vi "daq+.vi"() -> ()   [LabVIEW 2020]
uses:
  <vilib>/Instr/_visa.llb/VISA Configure Serial Port (Instr).vi
panel:
  in  "Tab Control":enum32{"CONFIG", "DASHBOARD"}(tab)
  in  "stop":bool
  in  "Baudios":u32=9600
  in  "Paridad":enum16{"None", "Odd", "Even", "Mark", "Space"}(ring)
  in  "Puerto COM":refnum<visa-resource-name>
  out "ADC-dsPIC33FJ32MC202":dbl[](array[slide]) scale=0.0..4095.0
  in  "LED1":bool
  in  "LED2":bool
  in  "LED3":bool
  in  "LED4":bool
  out "error out":errorcluster
  out "VISA resource name out":refnum<visa-resource-name>
  out "read buffer":string
  # "CURSO DSPIC Y SUS APLICACIONES\nCLASE 5"
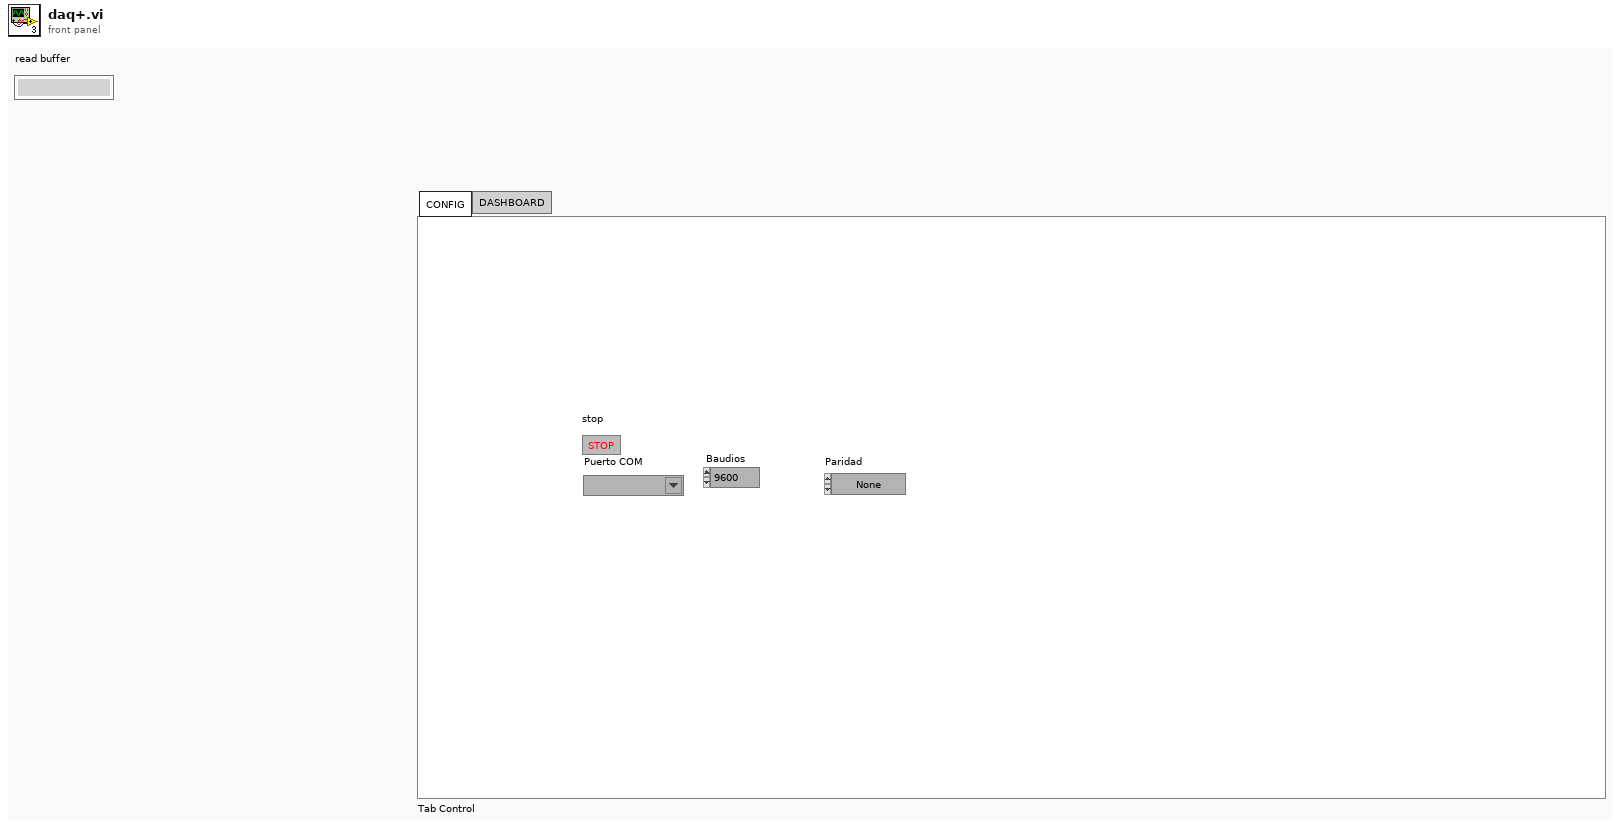
[diagram p1: front panel]
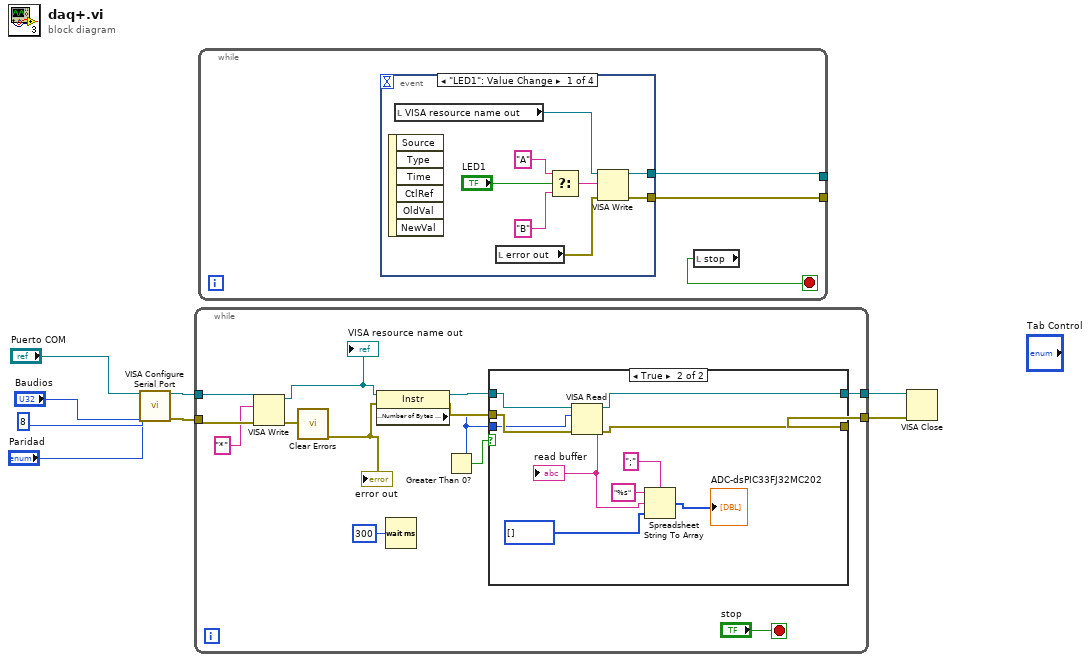
[diagram p0: block diagram]
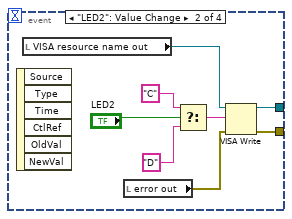
[diagram p2: hidden frame]
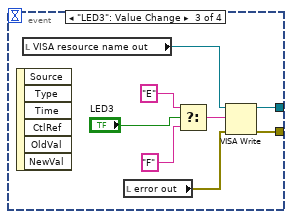
[diagram p3: hidden frame]
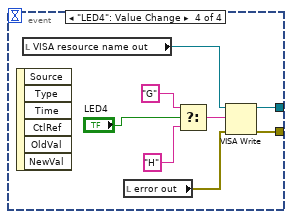
[diagram p4: hidden frame]
diagram:
  n1 = call-poly "VISA Configure Serial Port"("VISA resource name"="Puerto COM", "baud rate (9600)"="Baudios", "data bits (8)"=u16 8, "parity (0:none)"="Paridad") -> ("VISA resource name out"=w4:refnum<visa-resource-name>, "error out"=w3:errorcluster)  [unwired: 10 in]
  n2 = while {
    tunnel: w4 -> [w21]
    tunnel: w3 -> [w20]
    tunnel: [w14] -> w2
    tunnel: [w12] -> w1
    stop <- "stop" stop-if-true
    n3 = VISA Write(VISA resource name=w21, write buffer="*", error in (no error)=w20) -> (VISA resource name out=w9:refnum<visa-resource-name>, error out=w10:errorcluster)  [unwired: 1 out]
    "VISA resource name out" <- w9
    n4 = call <vilib>:"Clear Errors.vi"("error in (no error)"=w10) -> ("error out"=w11:errorcluster)  [unwired: 5 in, 1 out]
    "error out" <- w11
    n5 = property class="Instr"(reference=w9, error in=w11) -> (reference out=w17:refnum<visa-resource-name>, error out=w16:errorcluster, "Serial Settings:Number of Bytes at Serial Port"=w15:u32)
    n6 = Wait (ms)(milliseconds to wait=u32 300) -> ()  [unwired: 1 out]
    n7 = Greater Than 0?(x=w15) -> (x > 0?=w18:bool)
    n8 = case shown="True" w18 {
      tunnel: w17 -> [w24 w34]
      tunnel: w16 -> [w23 w33]
      tunnel: w15 -> [_ w32]
      tunnel: [w24 w26] -> w14
      tunnel: [w23 w25] -> w12
      frame False {
      }
      frame True {
        n9 = VISA Read(VISA resource name=w34, byte count=w32, error in (no error)=w33) -> (VISA resource name out=w26:refnum<visa-resource-name>, read buffer=w29:string, error out=w25:errorcluster)  [unwired: 1 out]
        "read buffer" <- w29
        n10 = Spreadsheet String To Array(delimiter (Tab)=";", format string="%s", spreadsheet string=w29, array type (2D Dbl)=i32[] []) -> (array=→"ADC-dsPIC33FJ32MC202":i32[])
      }
    }
  }
  n11 = while {
    tunnel: [w37] -> _
    tunnel: [w36] -> _
    stop <- w35 stop-if-true
    n12 = event shown="[0] \"LED1\": Value Change" {
      selector: _ -> [_ _ _ _]
      dyn-events: _ -> [_ _ _ _]
      timeout: _ -> [_ _ _ _]
      tunnel: [w39 w48 w56 w65] -> w37
      tunnel: [w38 w47 w55 w64] -> w36
      event "LED1": Value Change {
        n13 = event-data() -> ()  [unwired: 1 in, 6 out]
        n14 = local read "VISA resource name out"() -> (w41:refnum<visa-resource-name>)
        n15 = local read "error out"() -> (w40:errorcluster)
        n16 = Select(t="A", s="LED1", f="B") -> (s? t:f=w42:string)
        n17 = VISA Write(VISA resource name=w41, write buffer=w42, error in (no error)=w40) -> (VISA resource name out=w39:refnum<visa-resource-name>, error out=w38:errorcluster)  [unwired: 1 out]
      }
      event "LED2": Value Change {
        n18 = event-data() -> ()  [unwired: 1 in, 6 out]
        n19 = local read "VISA resource name out"() -> (w50:refnum<visa-resource-name>)
        n20 = local read "error out"() -> (w49:errorcluster)
        n21 = Select(t="C", s="LED2", f="D") -> (s? t:f=w51:string)
        n22 = VISA Write(VISA resource name=w50, write buffer=w51, error in (no error)=w49) -> (VISA resource name out=w48:refnum<visa-resource-name>, error out=w47:errorcluster)  [unwired: 1 out]
      }
      event "LED3": Value Change {
        n23 = event-data() -> ()  [unwired: 1 in, 6 out]
        n24 = local read "VISA resource name out"() -> (w58:refnum<visa-resource-name>)
        n25 = local read "error out"() -> (w57:errorcluster)
        n26 = Select(t="E", s="LED3", f="F") -> (s? t:f=w59:string)
        n27 = VISA Write(VISA resource name=w58, write buffer=w59, error in (no error)=w57) -> (VISA resource name out=w56:refnum<visa-resource-name>, error out=w55:errorcluster)  [unwired: 1 out]
      }
      event "LED4": Value Change {
        n28 = event-data() -> ()  [unwired: 1 in, 6 out]
        n29 = local read "VISA resource name out"() -> (w67:refnum<visa-resource-name>)
        n30 = local read "error out"() -> (w66:errorcluster)
        n31 = Select(t="G", s="LED4", f="H") -> (s? t:f=w68:string)
        n32 = VISA Write(VISA resource name=w67, write buffer=w68, error in (no error)=w66) -> (VISA resource name out=w65:refnum<visa-resource-name>, error out=w64:errorcluster)  [unwired: 1 out]
      }
    }
    n33 = local read "stop"() -> (w35:bool)
  }
  n34 = VISA Close(VISA resource name=w2, error in (no error)=w1) -> ()  [unwired: 1 out]
